vi "MF -Motor off.vi"(4 "error in":errorcluster, 5 "Action":bool, 6 "Axis #":i8=1 min=1 max=6 step=1, 7 "Address / Port":i16=1 min=1 max=31 step=1) -> (0 "error out":errorcluster, 1 "Motor power\nStatus - read":string, 2 "Axis # dup":i8=1 min=1 max=6 step=1, 3 "Address / Port dup":i16)   [LabVIEW 2014]
panel:
  # "Read"
  # "Write"
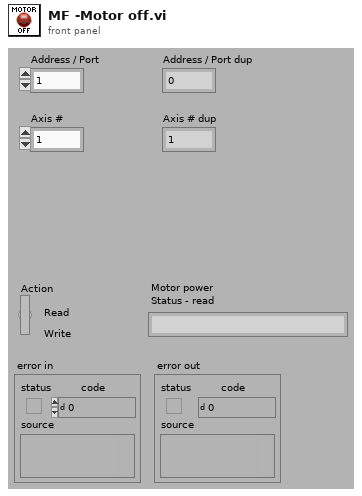
[diagram p1: front panel]
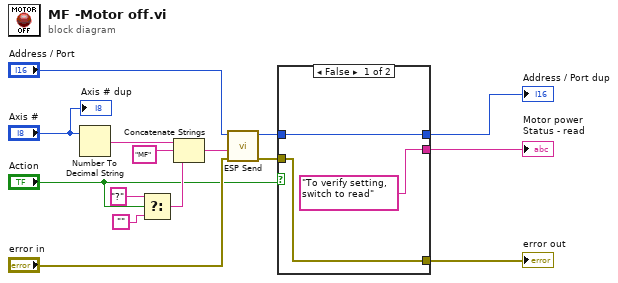
[diagram p0: block diagram]
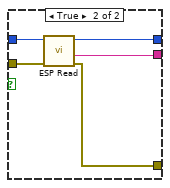
[diagram p2: hidden frame]
diagram:
  n1 = Number To Decimal String(number="Axis #") -> (decimal integer string=w14:string)  [unwired: 1 in]
  n2 = Select(t="?", s="Action", f="") -> (s? t:f=w11:string)
  n3 = Concatenate Strings(w14, "MF" ("Substring"), w11) -> (w12:string)
  n4 = call "ESP Send.vi"("error in"="error in", "Command String"=w12, "Address / Port"="Address / Port") -> ("error out"=w6:errorcluster, "Address / Port dup"=w2:i16)  [unwired: 3 in]
  n5 = case shown="False" "Action" {
    tunnel: w2 -> [w16 w23]
    tunnel: w6 -> [w18 w22]
    tunnel: [w18 w21] -> w5
    tunnel: ["To verify setting, switch to read" w20] -> w3
    tunnel: [w16 w19] -> w1
    frame False {
    }
    frame True {
      n6 = call "ESP Read.vi"("error in"=w22, "Address / Port"=w23) -> ("error out"=w21:errorcluster, "Response String"=w20:string, "Address / Port dup"=w19:i16)  [unwired: 3 in]
    }
  }
  "error out" <- w5
  "Motor power\nStatus - read" <- w3
  "Address / Port dup" <- w1
  "Axis # dup" <- "Axis #"
